vi "TrackerMain.vi"() -> (0 "Section list":i32[](array[numeric]))   [LabVIEW 2011]
uses:
  qtrk/QTrk.llb/QTrkZCommandType.ctl
  Typedefs/CmdEnum_UserInterfaceCmd.ctl
  qtrk/QTrk.llb/ResultManagerConfig.ctl
  qtrk/QTrk.llb/XYZf.ctl
  Camera/CIGrabParams.ctl
  qtrk/QTrk.llb/QTrkInstance.ctl
  Typedefs/TrackingConfigType.ctl
  qtrk/QTrk.llb/QTrkLocalizationType.ctl
  qtrk/QTrk.llb/ResultManagerInstance.ctl
  Camera/CIGrabControlMsg.ctl
  Camera/CIGrabControlMsgEnum.ctl
  ExperimentProgram/ExProgCommandEnumType.ctl
  GlobalVariables.vi
panel:
  out "Lost frames":i32
  in  "Offset factor":dbl=1.0
  in  "Gain factor":dbl=1.0
  out "Corner-based bead pos (out)":cluster{"X":i32, "Y":i32}[](array[cluster])
  in  "Close dialog":bool
  out "Framerate":i32
  out "Localizations done":i32
  out "Captured frames":i32
  out "Tracker internal profiling info":string
  out "Tracking queue %":i32
  out "[base]\\traces\\[expname].txt":path
  out "[base]\\traces\\[expname]_motors.txt":path
  out "Saved frames":i32
  out "Time(ms)":dbl
  out "script ended?":bool
  out "Instruction index":i32
  in  "End experiment":bool
  out "Frames complete":i32
  # "Running experiment"
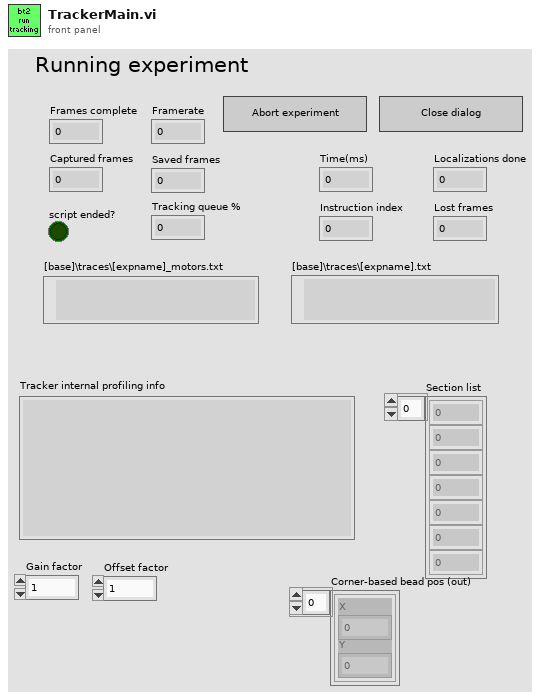
[diagram p1: front panel]
types:
  T1 = typedef "QTrkZCommandType.ctl" = enum16{"Nothing", "ComputeZ", "BuildRadialZLUT", "BuildImageZLUT", "RadialZLUT+ImageZLUT"}
  T2 = typedef "MeasureConfigType.ctl" = cluster{"Bead locations":cluster{"X":i32, "Y":i32}[], "ROI":i32, "Experiment base path":path, "Image output subdir":string, "Output mode":T3, "Traces output subdir":string, "QTrk Settings":T4, "Tracking Config":T5, "Experiment Name":string, "Program":T7, "ZLUT":sgl[][][], "Camera settings":T14, "Experiment Script":string, "Max frames in memory":i32, "Save traces as binary":bool, "Pixel Calibration Gain Image":string, "Pixel Calibration Offset Image":string, "Use pixel calibration images":bool, "Internal camera settings":string}
  T3 = typedef "MeasureConfigOutputMode.ctl" = enum16{"None", "Track", "SaveImages"}
  T4 = typedef "QTrkSettings.ctl" = cluster{"Image width":i32, "Image height":i32, "Number of threads (CPU based)":i32, "CUDA Device":i32, "COM Background correction factor":sgl, "ZLUT MinRadius":sgl, "ZLUT Radial sample density":sgl, "ZLUT Angular sample density":sgl, "ZLUT ROI Coverage":sgl, "QI Iterations":i32, "QI MinRadius":sgl, "QI Radial sample density":sgl, "QI Angular sample density":sgl, "QI ROI Coverage":sgl, "QI Angular Step \nIteration Factor":sgl, "XCOR Profile Length":i32, "XCOR Profile Width":i32, "XCOR Iterations":i32, "Gaussian 2D Fit Iterations":i32, "Gaussian 2D Sigma (pixels)":sgl}
  T5 = typedef "TrackingConfigType.ctl" = cluster{"Number of steps":i32, "ZLUT stepsize (um)":sgl, "Z correction factor":sgl, "Start piezo Z (um)":sgl, "Pixel size (nm)":sgl, "2D Localization Type":T6, "Z Command (None)":T1, "Z Piezo scale":bool}
  T6 = typedef "QTrkLocalizationType.ctl" = enum16{"Center-of-Mass", "1D Cross-Correlation", "Quadrant Interpolation", "Gaussian 2D MLE", "QI + ZLUTAlign", "ZLUTAlign"}
  T7 = typedef "ExperimentProgramType.ctl" = cluster{"Commands":T8[], "Motor Axis accuracy conditions":T11, "Axis flags":T13}
  T8 = typedef "ExProgCommandType.ctl" = cluster{"cmd":T9, "axis":T10, "value/pos":dbl, "speed":dbl, "name":string}
  T9 = typedef "ExProgCommandEnumType.ctl" = enum16{"wait", "move", "acquire", "idle", "rmove", "when", "section", "stop"}
  T10 = typedef "MotorAxisEnum.ctl" = enum16{"no axis", "magrot", "magpos", "px", "py", "pz", "camx", "camy"}
  T11 = typedef "MotorPosType.ctl" = cluster{"Magnet Z":dbl, "Magnet rotation":dbl, "Camera":T12, "Piezo XY":T12, "Piezo Z":dbl}
  T12 = typedef "XYf.ctl" = cluster{"X":sgl, "Y":sgl}
  T13 = typedef "MotorPosFlagsType.ctl" = cluster{"Magnet Z":bool, "Magnet rotation":bool, "Camera":cluster{"X":bool, "Y":bool}, "Piezo XY":cluster{"X":bool, "Y":bool}, "Piezo Z":bool}
  T14 = typedef "GenericCameraConfigType.ctl" = cluster{"Framerate (Hz)":i32, "Exposure time (us)":i32, "Image size":cluster{"Width":i32, "Height":i32}, "Number of buffers":i32}
  T15 = typedef "CmdEnum_UserInterfaceCmd.ctl" = enum32{"Idle (Use for default)", "ResultTracesUpdated", "MeasureConfigUpdated", "MeasureEnd", "MeasureStart"}
  T16 = typedef "ResultManagerConfig.ctl" = cluster{"Number of beads":i32, "Number of frame info columns":i32, "Result scaling":T17, "Result offset":T17, "Write Interval":i32, "Max frames in memory":i32, "Binary output (1/0)":i8}
  T17 = typedef "XYZf.ctl" = cluster{"X":sgl, "Y":sgl, "Z":sgl}
  T18 = typedef "ResultManagerInstance.ctl" = cluster{"InstancePtr":u64}
  T19 = typedef "QTrkInstance.ctl" = cluster{"QTrk Pointer":u64}
  T20 = typedef "CIGrabParams.ctl" = cluster{"Corner-based bead pos (out)":cluster{"X":i32, "Y":i32}[], "QTrk Instance":T19, "Tracking Config":T5, "ResultManager":T18, "Send to queue?":bool}
  T21 = typedef "CIGrabControlMsg.ctl" = cluster{"Msg":T22}
  T22 = typedef "CIGrabControlMsgEnum.ctl" = enum16{"Stop", "EnableTracking", "DisableTracking"}
  T23 = typedef "CameraInstance.ctl" = cluster{"VI refs":T24, "Camera state":variant}
  T24 = typedef "CameraInterface.ctl" = cluster{"Close":T25, "Get/Set generic config":T26, "Grab":T27, "Show Settings Dialog":T28, "AdjustBeadPos":T29, "Save/load camera settings":T30}
  T25 = typedef "CICloseType.ctl" = refnum<vi>
  T26 = typedef "CIGetSetGenericConfig.ctl" = refnum<vi>
  T27 = typedef "CIGrabType.ctl" = refnum<vi>
  T28 = typedef "CISettingsDlg.ctl" = refnum<vi>
  T29 = typedef "CIAdjustBeadPos.ctl" = refnum<vi>
  T30 = typedef "CISaveLoadSettings.ctl" = refnum<vi>
  T31 = typedef "ExProgState.ctl" = cluster{"Wanted Motorpos":T11, "Goal motorpos":T11, "Instruction":i32, "Speed":T11, "New instruction?":bool, "Instruction start time":dbl}
  T32 = typedef "QueueListType.ctl" = cluster{"Motor In":refnum<queue>, "User Interface Image View":refnum<queue>, "User Interface Camera Control":refnum<queue>, "User Interface Event Notifier":refnum<notifier>, "Initialized?":bool}
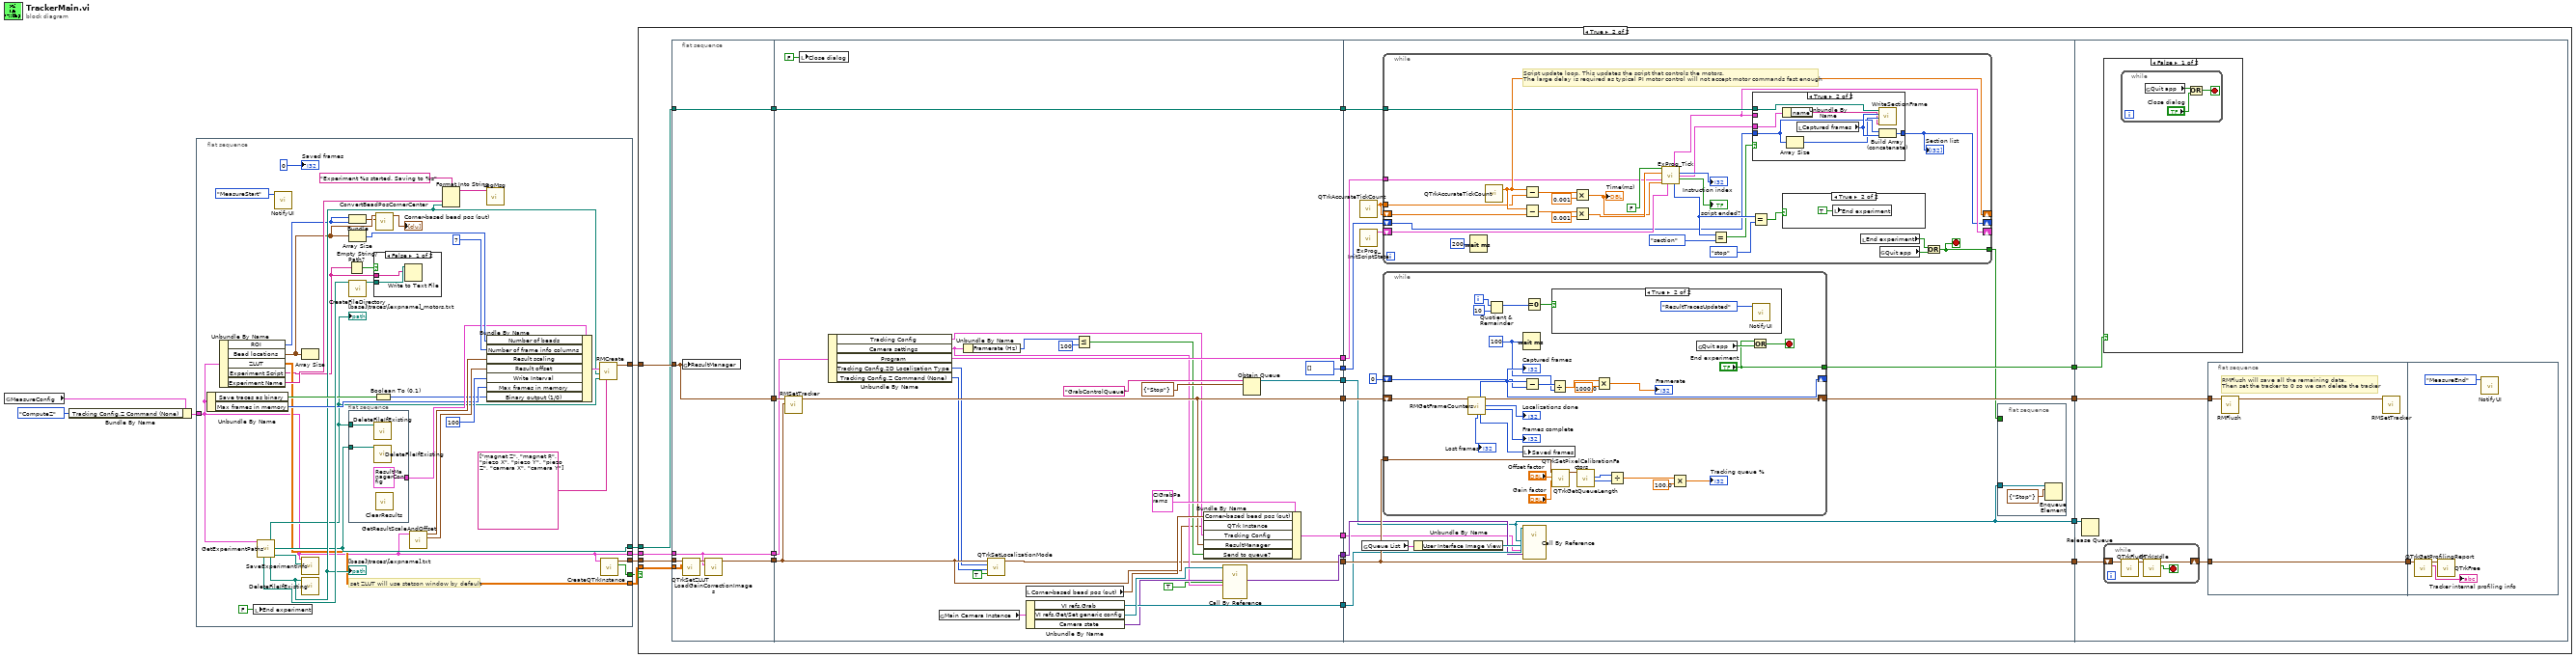
[diagram p0: block diagram]
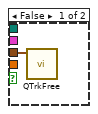
[diagram p2: hidden frame]
diagram:
  n1 = global read "GlobalVariables.vi" "MeasureConfig"() -> (w3:T2)
  n2 = Bundle By Name(cluster=w3, "Tracking Config.Z Command (None)"=QTrkZCommandType."ComputeZ") -> (w1:T2)
  n3 = flat-sequence {
    tunnel: [w20] -> w9
    tunnel: [w23] -> w7
    tunnel: [w22] -> w8
    tunnel: [w21] -> w6
    tunnel: [w14] -> w5
    tunnel: [w19] -> w4
    tunnel: w1 -> [w14]
    frame #0 {
      # "set ZLUT will use stetson window by default"
      n4 = Unbundle By Name(w14) -> ("Save traces as binary"=w30:bool, "Max frames in memory"=w31:i32)
      n5 = Unbundle By Name(w14) -> ("ROI"=w16:i32, "Bead locations"=w18:cluster{"X":i32, "Y":i32}[], "ZLUT"=w21:sgl[][][], "Experiment Script"=w13:string, "Experiment Name"=w27:string)
      n6 = local write "End experiment"(FALSE ("End experiment")) -> ()
      n7 = call "GetExperimentPaths.vi"("MeasureConfig"=w14) -> ("[base]\\traces\\[expname]_motors.txt"=w24:path, "[base]\\traces\\[expname]_sections.txt"=w23:path, "[base]\\[expname]_script.txt"=w41:path, "[base]\\traces\\[expname].txt/bin"=w26:path, "[base]\\traces\\[expname]_info.txt"=w42:path)  [unwired: 6 in, 4 out]
      "[base]\\traces\\[expname]_motors.txt" <- w24
      "[base]\\traces\\[expname].txt" <- w26
      n8 = call "NotifyUI.vi"("User Interface Commands"=CmdEnum_UserInterfaceCmd."MeasureStart") -> ()  [unwired: 11 in]
      n9 = Array Size(array=w18) -> ()  [unwired: 1 out]
      n10 = call "SaveExperimentInfo.vi"("File path"=w42, "MeasureConfig"=w14) -> ()  [unwired: 10 in]
      n11 = call "DeleteFileIfExisting.vi"("filename"=w26) -> ()  [unwired: 11 in]
      n12 = Empty String/Path?(string/path=w13) -> (empty?=w12:bool)
      n13 = flat-sequence {
        tunnel: [T16 {"Number of beads"=0, "Number of frame info columns"=0, "Result scaling"={"X"=0.0, "Y"=0.0, "Z"=0.0}, "Result offset"={"X"=0.0, "Y"=0.0, "Z"=0.0}, "Write Interval"=0, "Max frames in memory"=0, "Binary output (1/0)"=0} ("ResultManagerConfig")] -> w32
        tunnel: w24 -> [w47]
        tunnel: w23 -> [w46]
        frame #0 {
          n14 = call "DeleteFileIfExisting.vi"("filename"=w47) -> ()  [unwired: 11 in]
          n15 = call "DeleteFileIfExisting.vi"("filename"=w46) -> ()  [unwired: 11 in]
          n16 = call "ClearResults.vi"() -> ()  [unwired: 12 in]
        }
      }
      n17 = Bundle("ROI"=w16, "ROI"=w16) -> (w17:cluster{"ROI":i32, "ROI":i32})  [unwired: 1 in]
      n18 = Array Size(array=w18) -> (size(s)=w33:i32)
      n19 = call "CreateFileDirectory.vi"("filename"=w41) -> ("filename (copy)"=w40:path)  [unwired: 10 in]
      n20 = case shown="False" w12 {
        tunnel: w40 -> [w45 _]
        tunnel: w13 -> [w44 _]
        frame False {
          n21 = Write to Text File(file (use dialog)=w45, text=w44) -> ()  [unwired: 2 in, 3 out]
        }
        frame True {
        }
      }
      n22 = Boolean To (0,1)(Boolean=w30) -> (0, 1=w29:i16)
      n23 = call "ConvertBeadPosCornerCenter.vi"("ROI Size"=w17, "Center-based bead locations"=w18) -> ("Corner-based bead pos (out)"=→"Corner-based bead pos (out)":cluster{"X":i32, "Y":i32}[])  [unwired: 8 in, 1 out]
      n24 = call "GetResultScaleAndOffset.vi"("MeasureConfig"=w14) -> ("offset"=w35:cluster{dbl, dbl, "y":sgl}, "scale"=w36:cluster{sgl, sgl, sgl})  [unwired: 9 in]
      n25 = Format Into String(format string="Experiment %s started. Saving to %s", w27, w26) -> (resulting string=w25:string)  [unwired: 2 in, 1 out]
      n26 = call "LogMsg.vi"("msg"=w25) -> ()  [unwired: 11 in]
      n27 = Bundle By Name(cluster=w32, "Number of beads"=w33, "Number of frame info columns"=7, "Result scaling"=w36, "Result offset"=w35, "Write Interval"=100, "Max frames in memory"=w31, "Binary output (1/0)"=w29) -> (w38:T16)
      n28 = call "RMCreate.vi"("Frame info names"=string[] ["magnet Z", "magnet R", "piezo X", "piezo Y", "piezo Z", "camera X", "camera Y"], "frame info file"=w24, "output file"=w26, "ResultManagerConfig"=w38) -> ("ResultManager"=w22:T18)  [unwired: 7 in]
      n29 = call "CreateQTrkInstance.vi"("MeasureConfig"=w14) -> ("Go-ahead?"=w19:bool, "QTrk Instance"=w20:T19)  [unwired: 9 in]
      "Saved frames" <- 0 ("Saved frames")
    }
  }
  n30 = case shown="True" w4 {
    tunnel: w9 -> [w49 w62]
    tunnel: w8 -> [_ w61]
    tunnel: w7 -> [_ w60]
    tunnel: w6 -> [_ w59]
    tunnel: w5 -> [_ w58]
    frame False {
      n31 = call "QTrkFree.vi"("QTrk Instance"=w49) -> ()  [unwired: 6 in, 1 out]
    }
    frame True {
      n32 = flat-sequence {
        tunnel: [w73] -> w71
        tunnel: [w78] -> w70
        tunnel: [w77] -> w69
        tunnel: w62 -> [w75]
        tunnel: w61 -> [w78]
        tunnel: w60 -> [w77]
        tunnel: w59 -> [w76]
        tunnel: w58 -> [w72]
        tunnel: [w72] -> w57
        tunnel: w71 -> [w83]
        tunnel: [w103] -> w68
        tunnel: w70 -> [w107]
        tunnel: [w92] -> w67
        tunnel: [w82] -> w66
        tunnel: [i32[] [] ("initialized array")] -> w65
        tunnel: w69 -> [w105]
        tunnel: [w105] -> w64
        tunnel: [w90] -> w63
        tunnel: w57 -> [w104]
        tunnel: [w97] -> w53
        tunnel: [w95] -> w51
        tunnel: [w89] -> w50
        tunnel: w68 -> [w123]
        tunnel: w67 -> [w121]
        tunnel: w66 -> [w115]
        tunnel: w65 -> [w120]
        tunnel: w64 -> [w119]
        tunnel: w63 -> [w108]
        tunnel: [w117] -> w56
        tunnel: [w116] -> w55
        tunnel: [w115] -> w54
        tunnel: w53 -> [w114]
        tunnel: [w109] -> w52
        tunnel: w51 -> [w110]
        tunnel: w50 -> [w109]
        tunnel: w56 -> [w195]
        tunnel: w55 -> [w199]
        tunnel: w54 -> [w198]
        tunnel: w52 -> [w194]
        frame #0 {
          n33 = global write "GlobalVariables.vi" "ResultManager"(w78) -> ()
          n34 = call "QTrkSetZLUT.vi"("ZLUT"=w76, "QTrk Instance"=w75) -> ("QTrk Instance"=w74:T19)  [unwired: 8 in, 1 out]
          n35 = call "LoadGainCorrectionImages.vi"("MeasureConfig"=w72, "QTrk Instance in"=w74) -> ("QTrk Instance out"=w73:T19)  [unwired: 9 in]
        }
        frame #1 {
          n36 = call "RMSetTracker.vi"("QTrk Instance"=w83, "ResultManager"=w107) -> ("ResultManager (out)"=w92:T18)  [unwired: 8 in, 1 out]
          n37 = local write "Close dialog"(FALSE ("Close dialog")) -> ()
          n38 = Unbundle By Name(w104) -> ("Tracking Config"=w91:T5, "Camera settings"=w88:T14, "Program"=w103:T7, "Tracking Config.2D Localization Type"=w81:T6, "Tracking Config.Z Command (None)"=w80:T1)
          n39 = global read "GlobalVariables.vi" "Main Camera Instance"() -> (w99:T23)
          n40 = Unbundle By Name(w88) -> ("Framerate (Hz)"=w87:i32)
          n41 = call "QTrkSetLocalizationMode.vi"("Normalize profile"=TRUE, "Z Command"=w80, "2D Localization Type"=w81, "QTrk Instance"=w83) -> ("QTrk Instance"=w82:T19)  [unwired: 7 in]
          n42 = local read "Corner-based bead pos (out)"() -> (w93:cluster{"X":i32, "Y":i32}[])
          n43 = Unbundle By Name(w99) -> ("VI refs.Grab"=w97:T27, "VI refs.Get/Set generic config"=w98:T26, "Camera state"=w96:variant)
          n44 = Less Or Equal?(x=w87, y=100 ("x")) -> (x <= y?=w85:bool)
          n45 = Bundle By Name(cluster=T20 {"Corner-based bead pos (out)"=[], "QTrk Instance"={"QTrk Pointer"=0}, "Tracking Config"={"Number of steps"=0, "ZLUT stepsize (um)"=0.0, "Z correction factor"=0.0, "Start piezo Z (um)"=0.0, "Pixel size (nm)"=0.0, "2D Localization Type"=enum."Quadrant Interpolation", "Z Command (None)"=enum."Nothing", "Z Piezo scale"=FALSE}, "ResultManager"={"InstancePtr"=0}, "Send to queue?"=TRUE} ("TrackingParameters"), "Corner-based bead pos (out)"=w93, "QTrk Instance"=w83, "Tracking Config"=w91, "ResultManager"=w92, "Send to queue?"=w85) -> (w90:T20)
          n46 = call-by-ref "?"(reference=w98, "Set? (F)"=TRUE, "GenericCameraConfig"=w88, "Camera state"=w96) -> ("Camera state (out)"=w95:variant)  [unwired: 8 in, 3 out]
          n47 = Obtain Queue(name (unnamed)="GrabControlQueue", element data type=T21 {"Msg"=enum."Stop"} ("GrabControlMsg")) -> (queue out=w89:refnum<queue>)  [unwired: 3 in, 2 out]
        }
        frame #2 {
          n48 = call "QTrkAccurateTickCount.vi"() -> ("tick count (ms)"=w122:dbl)  [unwired: 2 in, 1 out]
          n49 = call "ExProg_InitScriptState.vi"() -> ("Script exec state out"=w124:T31)  [unwired: 11 in]
          n50 = global read "GlobalVariables.vi" "Queue List"() -> (w112:T32)
          n51 = while {
            shift-right: [w161] -> _
            shift-left: w124 -> [w180]
            shift-right: [w176] -> _
            shift-left: w122 -> [w181]
            tunnel: w123 -> [w160]
            tunnel: w122 -> [w175]
            shift-right: [w159] -> _
            shift-left: w120 -> [w163]
            tunnel: w119 -> [w162]
            tunnel: [w157] -> w113
            stop <- w157 stop-if-true
            # "Script update loop. This updates the script that controls the motors.\nThe large delay is required as typical PI motor control will not accept motor commands fast enough"
            n52 = Wait (ms)(milliseconds to wait=u32 200) -> ()  [unwired: 1 out]
            n53 = call "QTrkAccurateTickCount.vi"() -> ("tick count (ms)"=w176:dbl)  [unwired: 2 in, 1 out]
            n54 = Subtract(x=w176, y=w175) -> (x-y=w174:dbl)
            n55 = Subtract(x=w176, y=w181) -> (x-y=w171:dbl)
            n56 = Multiply(x=w174, y=0.001) -> (x*y=w169:dbl)
            "Time(ms)" <- w169
            n57 = Multiply(x=w171, y=0.001) -> (x*y=w170:dbl)
            n58 = call "ExProg_Tick.vi"("Simulation?"=FALSE, "Timestep (s)"=w170, "Program"=w160, "Current time (s)"=w169, "Script exec state in"=w180) -> ("Script exec state out"=w161:T31, "Instruction index"=→"Instruction index":i32, "Last instruction"=w158:T8, "script ended?"=→"script ended?":bool, "Last command"=w166:T9)  [unwired: 6 in]
            n59 = Equal?(x=w166, y=ExProgCommandEnumType."section") -> (x = y?=w164:bool)
            n60 = Equal?(x=w166, y=ExProgCommandEnumType."stop") -> (x = y?=w167:bool)
            n61 = case shown="True" w164 {
              tunnel: w163 -> [w185 w189]
              tunnel: [w185 w192] -> w159
              tunnel: w162 -> [_ w191]
              tunnel: w161 -> [_ _]
              tunnel: w158 -> [_ w186]
              frame False {
              }
              frame True {
                n62 = Unbundle By Name(w186) -> ("name"=w187:string)
                n63 = Array Size(array=w189) -> (size(s)=w188:i32)
                n64 = local read "Captured frames"() -> (w190:i32)
                n65 = call "WriteSectionFrame.vi"("section name"=w187, "section index"=w188, "section frame"=w190, "[base]\\traces\\[expname]_sections.txt"=w191) -> ()  [unwired: 8 in]
                n66 = Build Array (concatenate)(w189, w190) -> (w192:i32[])
              }
            }
            "Section list" <- w159
            n67 = case shown="True" w167 {
              frame False {
              }
              frame True {
                n68 = local write "End experiment"(TRUE ("End experiment")) -> ()
              }
            }
            n69 = local read "End experiment"() -> (w184:bool)
            n70 = global read "GlobalVariables.vi" "Quit app"() -> (w183:bool)
            n71 = Or(x=w184, y=w183) -> (x .or. y?=w157:bool)
          }
          n72 = while {
            tunnel: ["End experiment"] -> w116
            tunnel: w115 -> [w131]
            shift-right: [w152] -> w117
            shift-left: w121 -> [w151]
            shift-right: [w138] -> _
            shift-left: 0 ("capturedFrames") -> [w137]
            i -> [w148]
            stop <- w154 stop-if-true
            w135 = u32 100 ("milliseconds to wait")
            n73 = call "RMGetFrameCounters.vi"("ResultManager"=w151) -> ("capturedFrames"=w138:i32, "ResultManager (out)"=w152:T18, "totalLocalizationsDone"=→"Localizations done":i32, "endFrame"=→"Frames complete":i32, "lostFrames"=→"Lost frames":i32, "lastSaveFrame"=w149:i32)  [unwired: 7 in, 2 out]
            "Captured frames" <- w138
            n74 = Quotient & Remainder(x=w148, y=10) -> (x-y*floor(x/y)=w146:i32)  [unwired: 1 out]
            n75 = Wait (ms)(milliseconds to wait=w135) -> ()  [unwired: 1 out]
            n76 = local write "Saved frames"(w149) -> ()
            n77 = Subtract(x=w138, y=w137) -> (x-y=w136:i32)
            n78 = Equal To 0?(x=w146) -> (x = 0?=w145:bool)
            n79 = Divide(x=w136, y=w135) -> (x/y=w134:dbl)
            n80 = case shown="True" w145 {
              frame False {
              }
              frame True {
                n81 = call "NotifyUI.vi"("User Interface Commands"=CmdEnum_UserInterfaceCmd."ResultTracesUpdated") -> ()  [unwired: 11 in]
              }
            }
            n82 = call "QTrkSetPixelCalibrationFactors.vi"("gainFactor (1)"="Gain factor", "offsetFactor (1)"="Offset factor", "QTrk Instance"=w131) -> ("QTrk Instance"=w128:T19)  [unwired: 7 in, 1 out]
            n83 = call "QTrkGetQueueLength.vi"("QTrk Instance"=w128) -> ("maxQueueLen"=w143:i32, "queue size"=w144:i32)  [unwired: 7 in, 2 out]
            n84 = Multiply(x=w134, y=1000.0) -> (x*y=→"Framerate":dbl)
            n85 = Divide(x=w144, y=w143) -> (x/y=w142:dbl)
            n86 = Multiply(x=w142, y=100.0) -> (x*y=→"Tracking queue %":dbl)
            n87 = global read "GlobalVariables.vi" "Quit app"() -> (w155:bool)
            n88 = Or(x="End experiment", y=w155) -> (x .or. y?=w154:bool)
          }
          n89 = Unbundle By Name(w112) -> ("User Interface Image View"=w111:refnum<queue>)
          n90 = call-by-ref "?"(reference=w114, "Camera data"=w110, "TrackingParameters"=w108, "Output Queue"=w111, "GrabControlQueue"=w109) -> ()  [unwired: 8 in, 3 out]
          n91 = flat-sequence {
            tunnel: w113 -> [_]
            tunnel: w109 -> [w126]
            frame #0 {
              n92 = Enqueue Element(queue=w126, element=T21 {"Msg"=enum."Stop"}) -> ()  [unwired: 2 in, 3 out]
            }
          }
        }
        frame #3 {
          n93 = Release Queue(queue=w194) -> ()  [unwired: 2 in, 3 out]
          n94 = case shown="False" w199 {
            frame False {
              n95 = while {
                stop <- w211 stop-if-true
                n96 = global read "GlobalVariables.vi" "Quit app"() -> (w213:bool)
                n97 = Or(x=w213, y="Close dialog") -> (x .or. y?=w211:bool)
              }
            }
            frame True {
            }
          }
          n98 = while {
            shift-right: [w210] -> w196
            shift-left: w198 -> [w208]
            stop <- w209 stop-if-true
            n99 = call "QTrkFlush.vi"("QTrk Instance"=w208) -> ("QTrk Instance (out)"=w207:T19)  [unwired: 9 in, 1 out]
            n100 = call "QTrkIsIdle.vi"("QTrk Instance"=w207) -> ("Currently idle?"=w209:bool, "QTrk Instance (out)"=w210:T19)  [unwired: 8 in, 1 out]
          }
          n101 = flat-sequence {
            tunnel: [w201] -> w197
            tunnel: w196 -> [w201]
            tunnel: w195 -> [w200]
            tunnel: w197 -> [w203]
            frame #0 {
              # "RMFlush will save all the remaining data.\nThen set the tracker to 0 so we can delete the tracker"
              n102 = call "RMFlush.vi"("ResultManager"=w200) -> ("ResultManager (out)"=w202:T18)  [unwired: 9 in, 1 out]
              n103 = call "RMSetTracker.vi"("ResultManager"=w202) -> ()  [unwired: 9 in, 2 out]
            }
            frame #1 {
              n104 = call "QTrkGetProfilingReport.vi"("QTrk Instance"=w203) -> ("report"=→"Tracker internal profiling info":string, "QTrk Instance (out)"=w206:T19)  [unwired: 9 in]
              n105 = call "QTrkFree.vi"("QTrk Instance"=w206) -> ()  [unwired: 6 in, 1 out]
              n106 = call "NotifyUI.vi"("User Interface Commands"=CmdEnum_UserInterfaceCmd."MeasureEnd") -> ()  [unwired: 11 in]
            }
          }
        }
      }
    }
  }
